vi "check numeric.vi"(11 "String":string) -> (3 "all numeric?":bool)   [LabVIEW 2020]
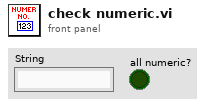
[diagram p1: front panel]
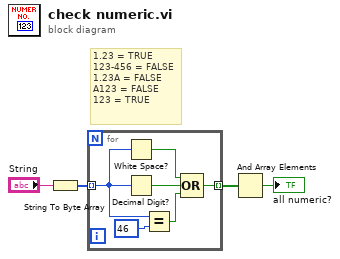
[diagram p0: block diagram]
diagram:
  # "1.23 = TRUE\n123-456 = FALSE\n1.23A = FALSE\nA123 = FALSE\n123 = TRUE"
  n1 = String To Byte Array(string="String") -> (unsigned byte array=w3:u8[])
  n2 = for {
    tunnel: w3 -> [w9] mode=indexing
    tunnel: [w5] -> w2 mode=indexing
    n3 = White Space?(1:w9) -> (0:w8:bool)
    n4 = Decimal Digit?(1:w9) -> (0:w7:bool)
    n5 = Equal?(x=w9, y=46) -> (x = y?=w6:bool)
    n6 = Compound Arithmetic op=OR(w8, w7, w6) -> (w5:bool)
  }
  n7 = And Array Elements(Boolean array=w2) -> (logical AND=→"all numeric?":bool)
